vi "Read Binary Configuration.vi"(7 "Type":T1, 8 "error in (no error)":errorcluster, 9 "Default If Not Found":variant, 10 "Name":string, 11 "database-configuration in":refnum<class "configuration-database.lvclass">) -> (0 "error out":errorcluster, 1 "Not Found?":bool, 2 "Value":variant, 3 "database-configuration out":refnum<class "configuration-database.lvclass">)   [LabVIEW 2020, in "configuration-database.lvlib" / "configuration-database.lvclass"]
uses:
  configuration-database.lvclass
  <vilib>/Utility/Data Type/Type Definitions/Data Type.ctl
  configuration-database.lvclass/configuration-database.ctl
  52724a25-5809-4a21-a2b8-aa90eb3c3470.vi
  <vilib>/Utility/error.llb/Error Cluster From Error Code.vi
  IConfigDBQueries/IConfigurationDatabaseQueries.lvclass
  externals/database-interface/IDatabase/IDatabase/IDatabase.lvclass
  <vilib>/Utility/Data Type/NI_Data Type.lvlib
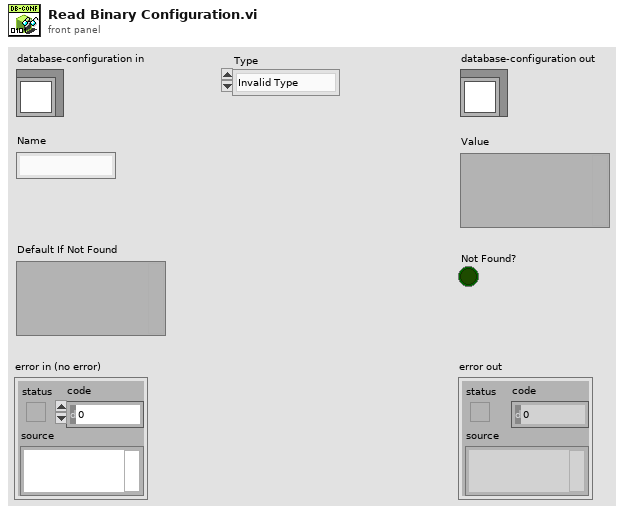
[diagram p1: front panel]
types:
  T1 = typedef "NI_Data Type.lvlib/Data Type.ctl" = enum8{"Invalid Type", "Void", "I8", "I16", "I32", "I64", "U8", "U16", "U32", "U64", "Single Float", "Double Float", "Extended Float", "Single Complex", "Double Complex", "Extended Complex", "Enum U8", "Enum U16", "Enum U32", "Enum U64", "Single Float With Unit", "Double Float With Unit", "Extended Float With Unit", "Single Complex with Unit", "Double Complex with Unit", "Extended Complex with Unit", "Boolean", "String", "Path", "Picture", "Tag", "Array", "Cluster", "Variant", "LV Variant", "Waveform", "Timestamp", "Digital Waveform", "Digital Data", "ExpressData", "Refnum", "External Data", "VI", "Poly VI", "LabVIEW Class Instance", "Fixed Point", "Set Collection", "Map Collection"}
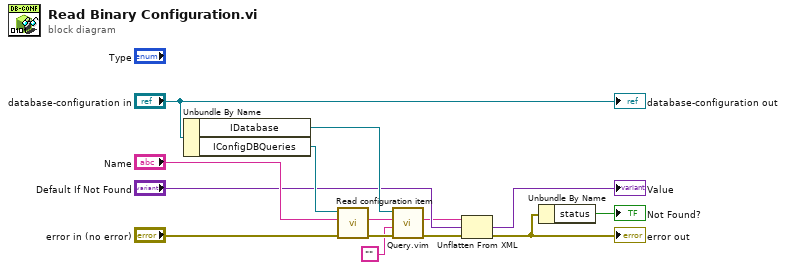
[diagram p0: block diagram]
diagram:
  n1 = Unbundle By Name("database-configuration in") -> ("IDatabase"=w12:refnum<class "IDatabase.lvclass">, "IConfigDBQueries"=w13:refnum<class "IConfigurationDatabaseQueries.lvclass">)
  n2 = call-dynamic "Read configuration item.vi"("error in (no error)"="error in (no error)", "configuration item"="Name", "IConfigDBQueries in"=w13) -> ("error out"=w11:errorcluster, "result"=w10:string)  [unwired: 7 in]
  n3 = call "Query.vim"("error in (no error)"=w11, "Type and Default"="", "Query string"=w10, "IDatabase in"=w12) -> ("error out"=w5:errorcluster, "Result"=w2:string)  [unwired: 5 in, 1 out]
  n4 = Unflatten From XML(xml string=w2, type="Default If Not Found", error in (no error)=w5) -> (value=→"Value":variant, error out=w4:errorcluster)
  "error out" <- w4
  n5 = Unbundle By Name(w4) -> ("status"=→"Not Found?":bool)
  "database-configuration out" <- "database-configuration in"
